vi "CreatePlots.vi"(7 "Main Graph":refnum<vi>, 8 "Error In":errorcluster, 9 "Sensors":u16(ring) items=["dwutlenek azotu", "ozon"], 10 "Plot data In":cluster{"Dates":timestamp[], "Values":dbl[]}, 11 "Prog data In":T1={"Station"=[], "Sensor List"=[], "Sensor Id"=[], "Parameters"=["PM10", "PM2.5", "ozon", "dwutlenek azotu", "dwutlenek siarki", "benzen", "tlenek węgla"], "Values"=[110, 75, 180, 200, 350, 21, 15]}) -> (0 "Error Out":errorcluster, 2 "XY Plots":cluster{"Dates":timestamp[], "Values":dbl[]}[](array[cluster]))   [LabVIEW 2020]
doc: "Based on sensor data makes threshold line and prepare all to XY graph format."
uses:
  Ctrls/ProgData.ctl
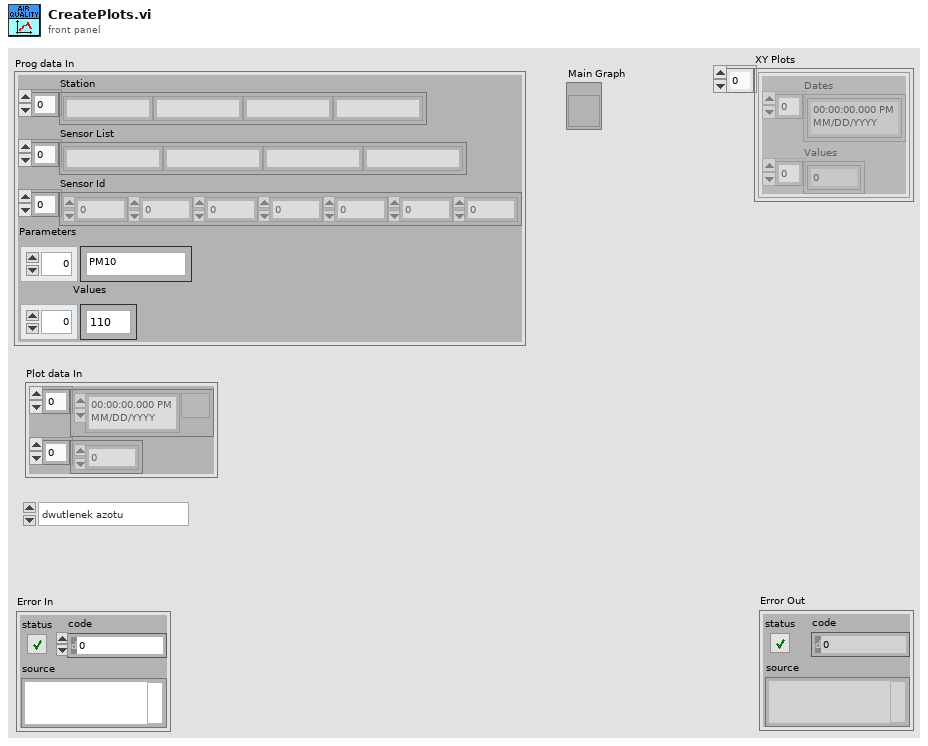
[diagram p1: front panel]
types:
  T1 = typedef "ProgData.ctl" = cluster{"Station":string[], "Sensor List":string[], "Sensor Id":dbl[], "Parameters":string[], "Values":i32[]}
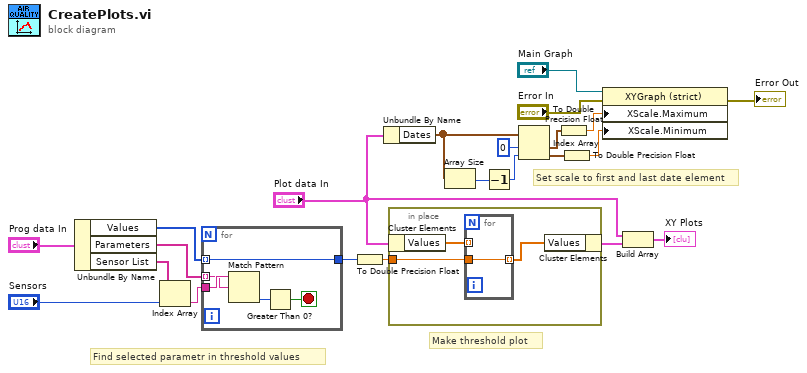
[diagram p0: block diagram]
diagram:
  # "Find selected parametr in threshold values"
  # "Make threshold plot"
  # "Set scale to first and last date element"
  n1 = Unbundle By Name("Prog data In") -> ("Values"=w20:i32[], "Parameters"=w21:string[], "Sensor List"=w15:string[])
  n2 = Index Array(array=w15, index="Sensors") -> (element=w13:string)
  n3 = for {
    tunnel: w13 -> [w24]
    tunnel: w21 -> [w23] mode=indexing
    tunnel: w20 -> [w25] mode=indexing
    tunnel: [w25] -> w19
    stop <- w26 stop-if-true
    n4 = Match Pattern(string=w24, regular expression=w23) -> (offset past match=w27:i32)  [unwired: 1 in, 3 out]
    n5 = Greater Than 0?(x=w27) -> (x > 0?=w26:bool)
  }
  n6 = To Double Precision Float(number=w19) -> (double precision float=w18:dbl)
  n7 = Unbundle By Name("Plot data In") -> ("Dates"=w9:timestamp[])
  n8 = in-place {
    in-place-border: w18 -> [w29]
    n9 = in-place-cluster #1("Plot data In") -> ("Values"=w30:dbl[])
    n10 = for {
      tunnel: w30 -> [_] mode=indexing
      tunnel: w29 -> [w31]
      tunnel: [w31] -> w28 mode=indexing
    }
    n11 = in-place-cluster #1("Values"=w28) -> (w16:cluster{"Dates":timestamp[], "Values":dbl[]})
  }
  n12 = Array Size(array=w9) -> (size(s)=w8:i32)
  n13 = Decrement(x=w8) -> (x-1=w7:i32)
  n14 = Index Array(array=w9, index #1=0 ("index"), index #2=w7) -> (element #1=w5:timestamp, element #2=w3:timestamp)
  n15 = To Double Precision Float(number=w5) -> (double precision float=w4:dbl)
  n16 = To Double Precision Float(number=w3) -> (double precision float=w2:dbl)
  n17 = property class="XYGraph (strict)"(reference="Main Graph", error in="Error In", "XScale.Maximum"=w4, "XScale.Minimum"=w2) -> (error out=→"Error Out":errorcluster)  [unwired: 1 out]
  n18 = Build Array("Plot data In", w16) -> (→"XY Plots":cluster{"Dates":timestamp[], "Values":dbl[]}[])
